vi "Vision Processing.vi"() -> ()   [LabVIEW 2015]
uses:
  <vilib>/Rock Robotics/WPI/Camera/WPI_CameraImageSize.ctl
  Vision Support Code/Camera Types.ctl
  <vilib>/userdefined/High Color/IMAQdx.ctl
  <vilib>/vision/driver/IMAQdx.llb/IMAQdx Camera Control Mode.ctl
  Robot Global Data.vi
  <vilib>/vision/NI_Vision_Development_Module.lvlib
  <vilib>/vision/driver/NI_Vision_Acquisition_Software.lvlib
panel:
  in  "Goal Width":dbl
  in  "Center Right":dbl
  in  "Center Left":dbl
  in  "Maximum Shooting Distance":dbl
  in  "Distance Method":u16(ring)=2 items=["Default", "Center Calculations", "Hybrid", "Ratios"]
  in  "Camera Distance\nfrom Ground (in)":dbl
  out "More Detection":T1(array[cluster])
  in  "Mask Color":i32=1
  in  "Y Res":i32=240
  in  "X Res":i32=320
  in  "Session In":T2="cam6"
  in  "Camera Type":T3=enum."MS HD3000 640x480"
  in  "error in (no error)":errorcluster
  in  "Image Size":T4=enum."320x240"
  out "ms to process":u32
  in  "LED Color":T5={"Hue"={91.12518353230051, 179.40124989546868}, "Sat"={197.32142857142858, 255.0}, "Val"={182.14285714285714, 255.0}} {"Hue" scale=0.0..255.0 scale format="%#_3g"}
  out "Qualified Particles":i32
  in  "Score Threshold":dbl=75.0
  in  "Aspect Fudge Factor":dbl=1.0
  in  "Min Score Threshold":i32=75
  in  "Emphasize Limit Tests":bool=TRUE
  out "Masked":T6(plugin-control)
  in  "Display Mask":bool=TRUE
  out "Original Image":T6(plugin-control)
  in  "Display Original":bool=TRUE
  out "Sorted Particle Scores":T7(array[cluster]) {"Moment Factor" format="%#_3g"; "Aspect Ratio" format="%#_3g"; "Area to CH" format="%#_3g"; "X" format="%#_3g"; "Y" format="%#_3g"}
  out "Highest Avg Score":dbl
  out "Detected Targets":T8(array[cluster]) {"Normalized Rect"."Numeric 5" format="%#_2g"; "Normalized Rect"."Numeric 3" format="%#_2g"; "Normalized Rect"."Numeric 2" format="%#_2g"; "Normalized Rect"."Numeric" format="%#_2g"}
  out "fps":dbl
  # "Density Profile"
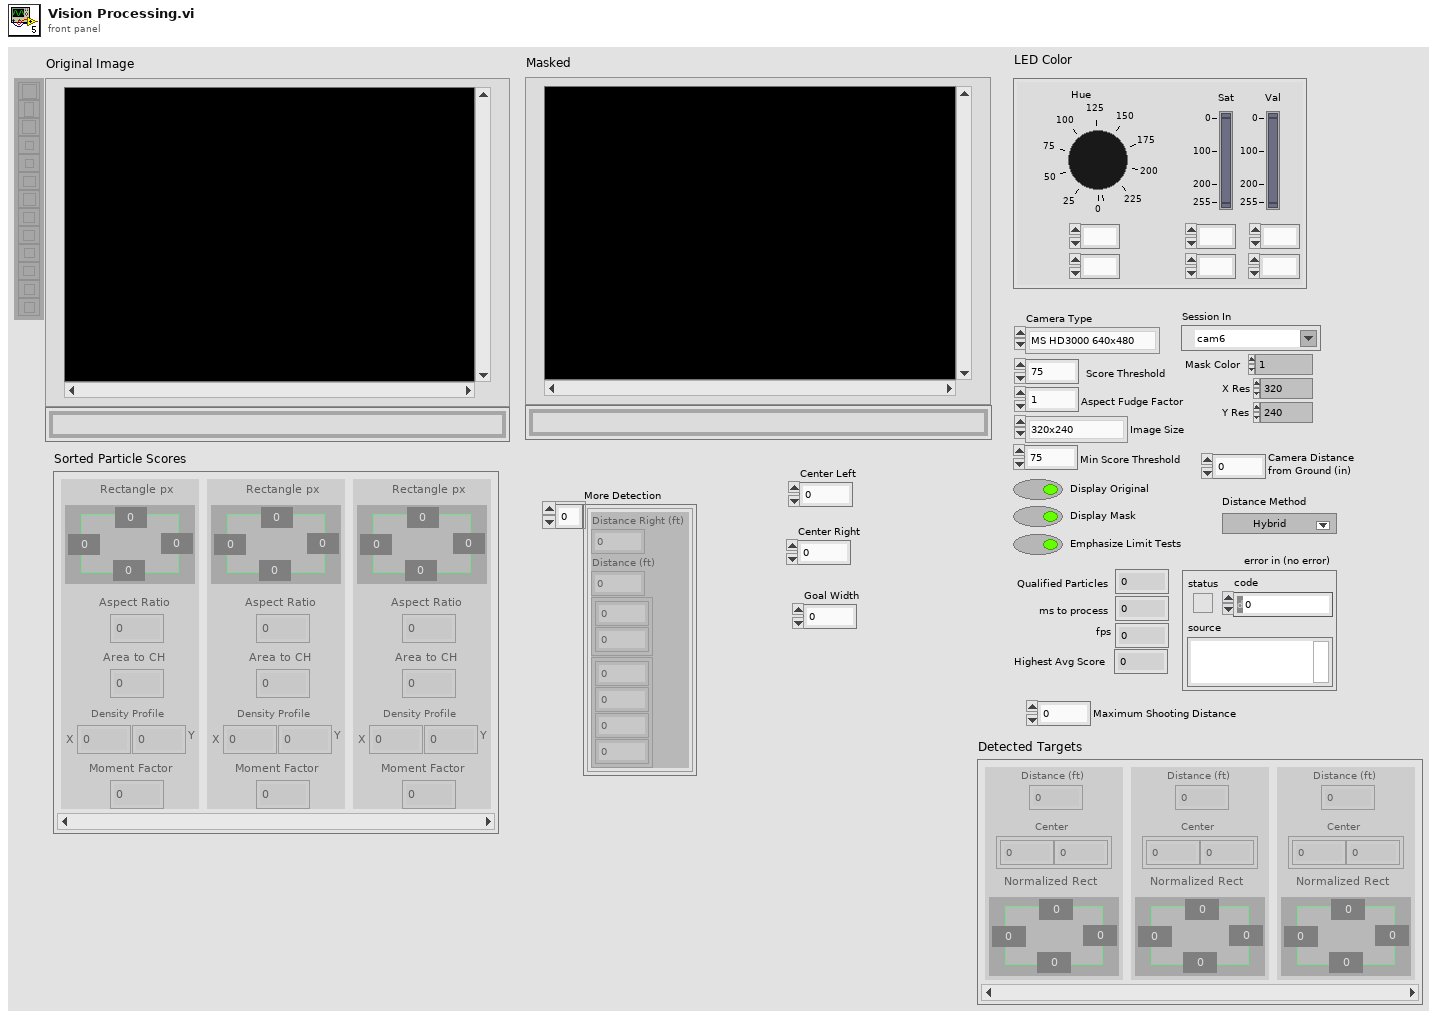
[diagram p1: front panel]
types:
  T1 = cluster{"Distance Right (ft)":dbl, "Distance (ft)":dbl, cluster{dbl, dbl}, cluster{dbl, dbl, dbl, dbl}}[]
  T2 = typedef "IMAQdx.ctl" = refnum<k21>
  T3 = typedef "Camera Types.ctl" = enum16{"206", "1011", "1013", "MS HD3000 square", "MS HD3000 640x480"}
  T4 = typedef "WPI_CameraImageSize.ctl" = enum16{"640x480", "320x240", "160x120", "Custom"}
  T5 = cluster{"Hue":cluster{dbl, dbl}, "Sat":cluster{dbl, dbl}, "Val":cluster{dbl, dbl}}
  T6 = typedef "IMAQ Image.ctl" = refnum<image>
  T7 = cluster{"Rectangle px":cluster{"Numeric":dbl, "Numeric 2":dbl, "Numeric 3":dbl, "Numeric 5":dbl}, "Aspect Ratio":dbl, "Area to CH":dbl, "X":dbl, "Y":dbl, "Moment Factor":dbl}[]
  T8 = cluster{"Distance (ft)":dbl, "Center":cluster{dbl, dbl}, "Normalized Rect":cluster{"Numeric":dbl, "Numeric 2":dbl, "Numeric 3":dbl, "Numeric 5":dbl}}[]
  T9 = typedef "Image Type" = u32
  T10 = typedef "NI_Vision_Acquisition_Software.lvlib/IMAQdx Camera Control Mode.ctl" = enum32{"Controller", "Listener"}
  T11 = typedef "Particle Parameters" = i32
  T12 = cluster{"Bounding box":cluster{"left":dbl, "top":dbl, "right":dbl, "bottom":dbl}, "Aspect Ratio":dbl, "Area to CH":dbl, "X Mask":dbl, "Y Mask":dbl, "Moment":dbl}[]
  T13 = cluster{"Numeric":dbl, "Numeric":dbl, dbl, dbl, "Numeric":dbl, "Numeric":dbl}[]
  T14 = cluster{"Rectangle":cluster{"Numeric":dbl, "Numeric 2":dbl, "Numeric 3":dbl, "Numeric 5":dbl}, "L":dbl, "Area to CH":dbl, "X":dbl, "Y":dbl, "Moment Factor":dbl}[]
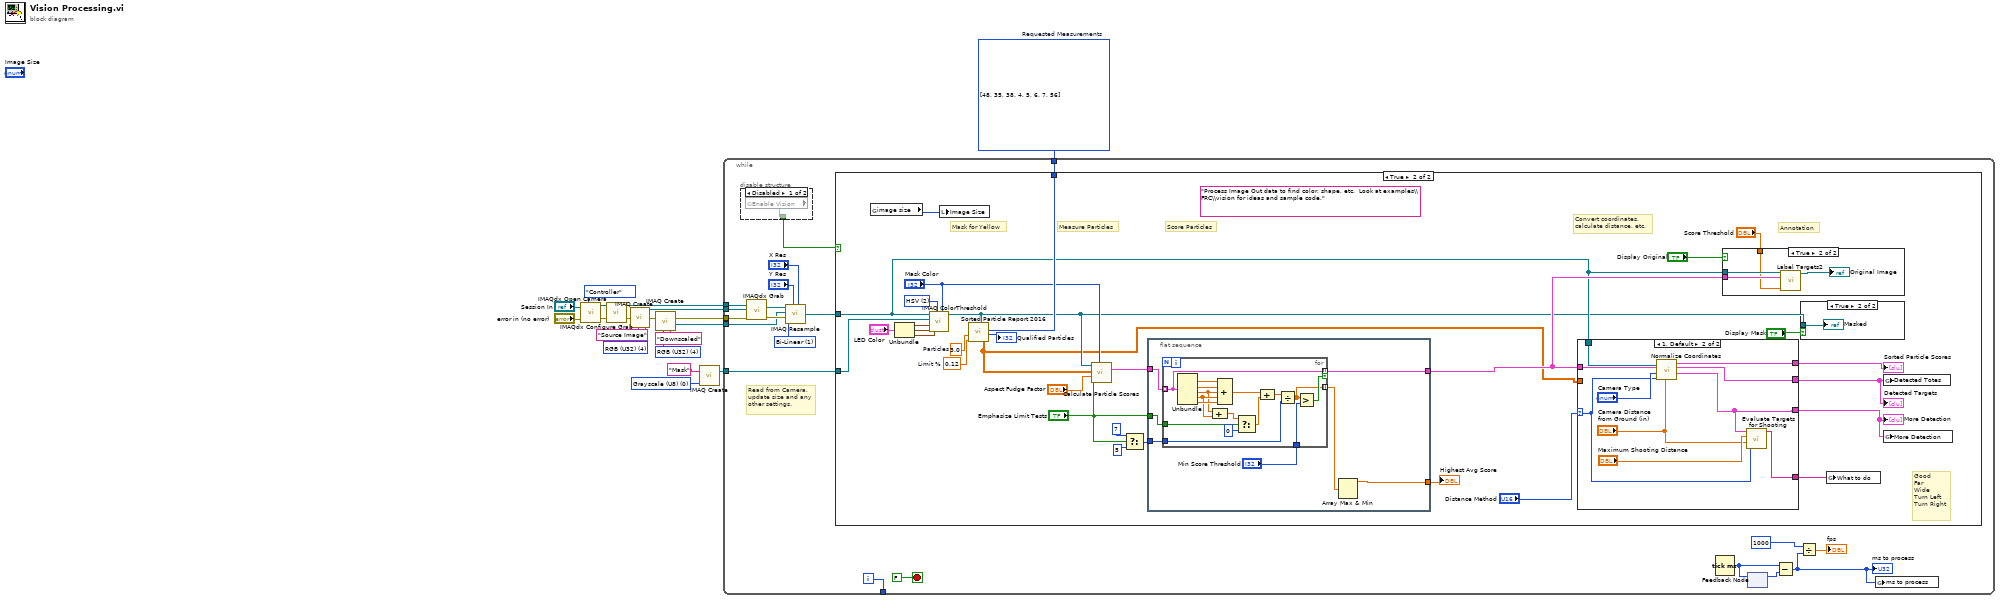
[diagram p0: block diagram]
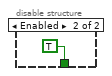
[diagram p2: hidden frame]
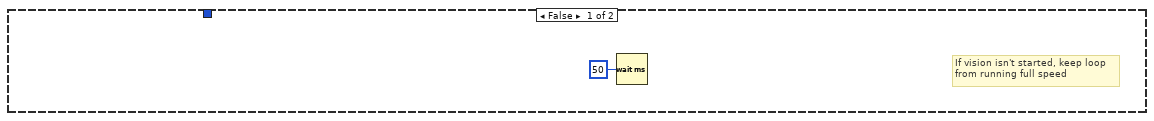
[diagram p3: hidden frame]
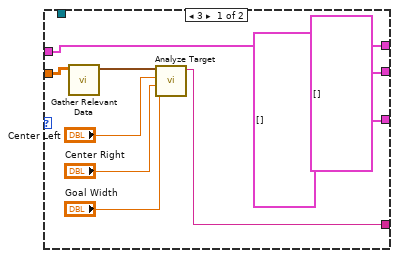
[diagram p4: hidden frame]
diagram:
  w9 = T9 4 items=["Grayscale (U8)", "Grayscale (I16)", "Grayscale (SGL)", "Complex (CSG)", "RGB (U32)", "HSL (U32)", "RGB (U64)", "Grayscale (U16)"] ("Image Type")
  w11 = T9 4 items=["Grayscale (U8)", "Grayscale (I16)", "Grayscale (SGL)", "Complex (CSG)", "RGB (U32)", "HSL (U32)", "RGB (U64)", "Grayscale (U16)"] ("Image Type")
  w17 = T11[] [48, 35, 38, 4, 5, 6, 7, 56] items=["Center of Mass X", "Center of Mass Y", "First Pixel X", "First Pixel Y", "Bounding Rect Left", "Bounding Rect Top", "Bounding Rect Right", "Bounding Rect Bottom", "Max Feret Diameter Start X", "Max Feret Diameter Start Y", "Max Feret Diameter End X", "Max Feret Diameter End Y", "Max Horiz. Segment Length Left", "Max Horiz. Segment Length Right", "Max Horiz. Segment Length Row", "-", "Bounding Rect Width", "Bounding Rect Height", "Bounding Rect Diagonal", "Perimeter", "Convex Hull Perimeter", "Holes' Perimeter", "Max Feret Diameter", "Equivalent Ellipse Major Axis", "Equivalent Ellipse Minor Axis", "Equivalent Ellipse Minor Axis (Feret)", "Equivalent Rect Long Side", "Equivalent Rect Short Side", "Equivalent Rect Diagonal", "Equivalent Rect Short Side (Feret)", "Average Horiz. Segment Length", "Average Vert. Segment Length", "Hydraulic Radius", "Waddel Disk Diameter", "-", "Area", "Holes' Area", "Particle & Holes' Area", "Convex Hull Area", "Image Area", "-", "Number of Holes", "Number of Horiz. Segments", "Number of Vert. Segments", "-", "Orientation", "Max Feret Diameter Orientation", "-", "% Area/Image Area", "% Area/(Particle & Holes' Area)", "Ratio of Equivalent Ellipse Axes", "Ratio of Equivalent Rect Sides", "-", "Elongation Factor", "Compactness Factor", "Heywood Circularity Factor", "Type Factor", "-", "Sum X", "Sum Y", "Sum XX", "Sum XY", "Sum YY", "Sum XXX", "Sum XXY", "Sum XYY", "Sum YYY", "-", "Moment of Inertia XX", "Moment of Inertia XY", "Moment of Inertia YY", "Moment of Inertia XXX", "Moment of Inertia XXY", "Moment of Inertia XYY", "Moment of Inertia YYY", "Norm. Moment of Inertia XX", "Norm. Moment of Inertia XY", "Norm. Moment of Inertia YY", "Norm. Moment of Inertia XXX", "Norm. Moment of Inertia XXY", "Norm. Moment of Inertia XYY", "Norm. Moment of Inertia YYY", "Hu Moment 1", "Hu Moment 2", "Hu Moment 3", "Hu Moment 4", "Hu Moment 5", "Hu Moment 6", "Hu Moment 7"]  # Requested Measurements
  w19 = T9 0 items=["Grayscale (U8)", "Grayscale (I16)", "Grayscale (SGL)", "Complex (CSG)", "RGB (U32)", "HSL (U32)", "RGB (U64)", "Grayscale (U16)"] ("Image Type")
  n1 = call <vilib>:"IMAQdx Open Camera.vi"("Camera Control Mode"=IMAQdx_Camera_Control_Mode."Controller", "error in"="error in (no error)", "Session In"="Session In") -> ("error out"=w14:errorcluster, "Session Out"=w16:T2)  [unwired: 7 in]
  n2 = call <vilib>:"IMAQdx Configure Grab.vi"("error in"=w14, "Session In"=w16) -> ("error out"=w13:errorcluster, "Session Out"=w7:T2)  [unwired: 8 in]
  n3 = call "IMAQ Create"("Image Name"="Source Image", "Image Type"=w11, "error in (no error)"=w13) -> ("New Image"=w4:T6, "error out"=w8:errorcluster)  [unwired: 2 in]
  n4 = call "IMAQ Create"("Image Name"="Downscaled", "Image Type"=w9, "error in (no error)"=w8) -> ("New Image"=w3:T6, "error out"=w5:errorcluster)  [unwired: 2 in]
  n5 = call "IMAQ Create"("Image Name"="Mask", "Image Type"=w19) -> ("New Image"=w18:T6)  [unwired: 2 in, 2 out]
  n6 = while {
    tunnel: w18 -> [w38]
    tunnel: w17 -> [w37]
    tunnel: [w34] -> _
    tunnel: w7 -> [w28]
    tunnel: w5 -> [w27]
    tunnel: w4 -> [w26]
    tunnel: w3 -> [w25]
    i -> [w34]
    stop <- FALSE stop-if-true
    w20 = u32 1 items=["Zero Order", "Bi-Linear", "Quadratic", "Cubic Spline"] ("Interpolation Type")
    # "Read from Camera,\nupdate size and any\nother settings."
    n7 = disable-structure shown="Disabled" {
      disable-tunnel: [w40 TRUE] -> w21
      frame Disabled {
        n8 = global read "Robot Global Data.vi" "Enable Vision"() -> (w40:bool)
      }
      frame Enabled {
      }
    }
    n9 = call <vilib>:"IMAQdx Grab.vi"("error in"=w27, "Image In"=w26, "Session In"=w28) -> ("error out"=w29:errorcluster, "Image Out"=w30:T6)  [unwired: 5 in, 2 out]
    n10 = call "IMAQ Resample"("X Resolution"="X Res", "Y Resolution"="Y Res", "error in (no error)"=w29, "Interpolation Type"=w20, "Image Dst"=w25, "Image Src"=w30) -> ("Image Dst Out"=w22:T6)  [unwired: 4 in, 1 out]
    n11 = case shown="True" w21 {
      tunnel: w38 -> [_ w73]
      tunnel: w37 -> [_ w59]
      tunnel: w22 -> [_ w52]
      frame False {
        # "If vision isn't started, keep loop\nfrom running full speed"
        n12 = Wait (ms)(milliseconds to wait=u32 50) -> ()  [unwired: 1 out]
      }
      frame True {
        w66 = u16 2 items=["RGB", "HSL", "HSV", "HSI"] ("Color Mode")
        (unwired) "Process Image Out data to find color, shape, etc.  Look at examples\\FRC\\vision for ideas and sample code."
        w58 = 0.12  # Limit %
        w57 = 3.0  # Particles
        # "Good\nFar\nWide\nTurn Left\nTurn Right"
        # "Measure Particles"
        # "Convert coordinates,\ncalculate distance, etc."
        # "Annotation"
        # "Score Particles"
        # "Mask for Yellow"
        n13 = global read "Robot Global Data.vi" "image size"() -> (w51:T4)
        n14 = Unbundle("LED Color") -> ("Hue"=w72:cluster{dbl, dbl}, "Sat"=w71:cluster{dbl, dbl}, "Val"=w70:cluster{dbl, dbl})
        n15 = call "IMAQ ColorThreshold"("Blue or Luma or Val or Inten Range"=w70, "Replace Value"="Mask Color", "Green or Sat Range"=w71, "Color Mode"=w66, "Red or Hue Range"=w72, "Image Dst"=w73, "Image Src"=w52) -> ("Image Dst Out"=w49:T6)  [unwired: 3 in, 1 out]
        n16 = local write "Image Size"(w51) -> ()
        n17 = call "Sorted Particle Report 2016.vi"("Min Area Size %"=w58, "Particle Count Limit"=w57, "Pixel Measurements"=w59, "Image in"=w49) -> ("Sorted Data"=w44:dbl[][], "Particles"=→"Qualified Particles":i32)
        n18 = call "Calculate Particle Scores.vi"("Pixel Value"="Mask Color", "Limit Tests?"="Emphasize Limit Tests", "Aspect Fudge Factor"="Aspect Fudge Factor", "Sorted Data"=w44, "Image in"=w49) -> ("Scores"=w56:T12)  [unwired: 6 in]
        n19 = Select(t=7, s="Emphasize Limit Tests", f=5) -> (s? t:f=w63:i32)
        n20 = flat-sequence {
          tunnel: w56 -> [w103]
          tunnel: w63 -> [w101]
          tunnel: [w104] -> w62
          tunnel: [w98] -> w53
          tunnel: "Emphasize Limit Tests" -> [w102]
          frame #0 {
            n21 = for {
              tunnel: w103 -> [w118] mode=indexing
              tunnel: [w118] -> w98 mode=indexing if=w117
              tunnel: [w116] -> w99 mode=indexing
              tunnel: w101 -> [w115]
              tunnel: "Min Score Threshold" -> [w114]
              tunnel: w102 -> [w107]
              n22 = Unbundle(w118) -> ("Aspect Ratio"=w120:dbl, "Area to CH"=w119:dbl, "X Mask"=w109:dbl, "Y Mask"=w110:dbl, "Moment"=w111:dbl)  [unwired: 1 out]
              n23 = Compound Arithmetic op=ADD(w109, w110) -> (w108:dbl)
              n24 = Compound Arithmetic op=ADD(w120, w119, w109, w110, w111) -> (w113:dbl)
              n25 = Select(t=w108, s=w107, f=0) -> (s? t:f=w106:dbl)
              n26 = Compound Arithmetic op=ADD(w113, w106) -> (w112:dbl)
              n27 = Divide(x=w112, y=w115) -> (x/y=w116:dbl)
              n28 = Greater?(x=w116, y=w114) -> (0:w117:bool)
            }
            n29 = Array Max & Min(array=w99) -> (max value=w104:dbl)  [unwired: 3 out]
          }
        }
        n30 = case shown="1, Default" "Distance Method" {
          selector: "Distance Method" -> [_ w84]
          tunnel: w53 -> [w76 w92]
          tunnel: w52 -> [_ w91]
          tunnel: [w76 w90] -> w48
          tunnel: [T8 [] ("Found Targets") w89] -> w47
          tunnel: [T1 [] ("Array") w87] -> w46
          tunnel: w44 -> [w82 _]
          tunnel: [w80 w83] -> w43
          frame 3 {
            n31 = call "Gather Relevant Data.vi"("Sorted Data"=w82) -> ("Relevant Data"=w81:T13)  [unwired: 10 in]
            n32 = call "Analyze Target.vi"("Goal Width"="Goal Width", "Center Right"="Center Right", "Center Left"="Center Left", "Relevant Data"=w81) -> ("What to do"=w80:string)  [unwired: 7 in]
          }
          frame 1, Default {
            n33 = call "Normalize Coordinates.vi"("Camera Distance\nfrom Ground (in)"="Camera Distance\nfrom Ground (in)", "Distance Method"=w84, "Camera Type"="Camera Type", "Targets"=w92, "Image in"=w91) -> ("Array"=w87:T1, "Found Targets"=w89:T8, "Sorted Scores"=w90:T14)  [unwired: 4 in]
            n34 = call "Evaluate Targets for Shooting.vi"("Distance Method"=w84, "Camera Distance\nfrom Ground (in)"="Camera Distance\nfrom Ground (in)", "Maximum Shooting Distance"="Maximum Shooting Distance", "More Detection"=w87) -> ("What to do"=w83:string)  [unwired: 6 in]
          }
        }
        "Sorted Particle Scores" <- w48
        "Detected Targets" <- w47
        "More Detection" <- w46
        n35 = case shown="True" "Display Original" {
          tunnel: w52 -> [_ w95]
          tunnel: w53 -> [_ w94]
          tunnel: "Score Threshold" -> [_ w93]
          frame False {
          }
          frame True {
            n36 = call "Label Targets2.vi"("Score Threshold"=w93, "Targets"=w94, "Image in"=w95) -> ("Image out"=→"Original Image":T6)  [unwired: 8 in]
          }
        }
        n37 = case shown="True" "Display Mask" {
          tunnel: w49 -> [_ w97]
          frame False {
          }
          frame True {
            "Masked" <- w97
          }
        }
        n38 = global write "Robot Global Data.vi" "What to do"(w43) -> ()
        n39 = global write "Robot Global Data.vi" "Detected Totes"(w47) -> ()
        n40 = global write "Robot Global Data.vi" "More Detection"(w46) -> ()
        "Highest Avg Score" <- w62
      }
    }
    n41 = Tick Count (ms)() -> (millisecond timer value=w35:u32)
    n42 = feedback-in #1(w35) -> ()
    n43 = feedback #1() -> (w36:u32)  [unwired: 1 in]
    n44 = Subtract(x=w35, y=w36) -> (x-y=w33:u32)
    "ms to process" <- w33
    n45 = Divide(x=1000 ("Brightness"), y=w33) -> (x/y=→"fps":dbl)
    n46 = global write "Robot Global Data.vi" "ms to process"(w33) -> ()
  }
